vi "Write User Events.vi"(8 "error in (no error)":errorcluster, 10 "User Events to TCP Engine":T1, 11 "SLL Easy API via TCP in":refnum<class "SLL Easy API via TCP.lvclass">) -> (0 "error out":errorcluster, 3 "SLL Easy API via TCP out":refnum<class "SLL Easy API via TCP.lvclass">)   [LabVIEW 2016, in "SLL Easy API via TCP.lvclass"]
uses:
  SLL Easy API via TCP.lvclass
  _Typedefs/User Events to TCP Engine.ctl
  _Typedefs/TCP Event Data.ctl
  SLL Easy API via TCP.lvclass/SLL Easy API via TCP.ctl
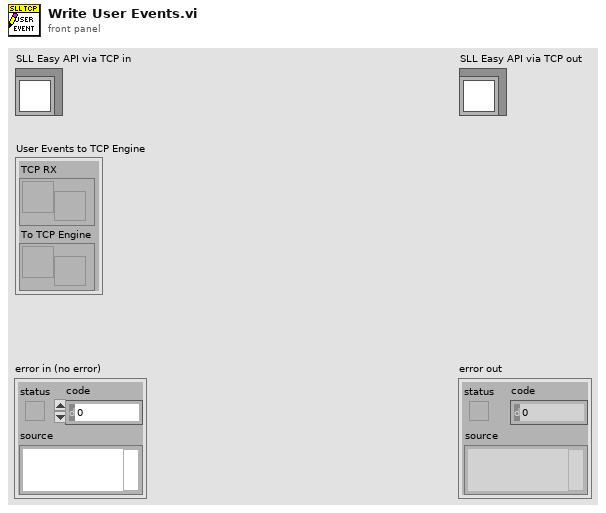
[diagram p1: front panel]
types:
  T1 = typedef "SLL Easy API via TCP.lvclass/User Events to TCP Engine.ctl" = cluster{"TCP RX":refnum<user-event>, "To TCP Engine":refnum<user-event>}
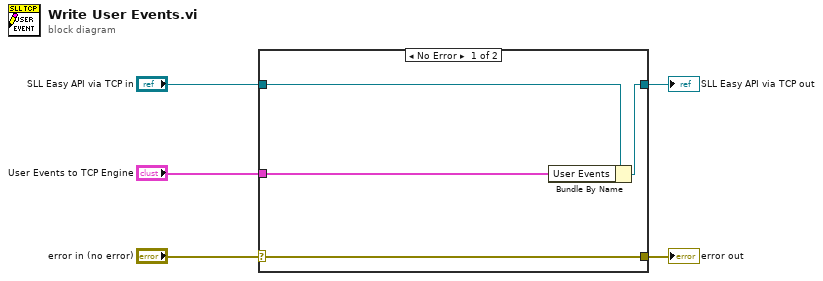
[diagram p0: block diagram]
diagram:
  n1 = case shown="No Error" "error in (no error)" {
    selector: "error in (no error)" -> [w9 w10]
    tunnel: [w9 w10] -> w4
    tunnel: [w7 w11] -> w2
    tunnel: "SLL Easy API via TCP in" -> [w8 w11]
    tunnel: "User Events to TCP Engine" -> [w6 _]
    frame No Error {
      n2 = Bundle By Name(cluster=w8, "User Events"=w6) -> (w7:refnum<class "SLL Easy API via TCP.lvclass">)
    }
    frame Error {
    }
  }
  "error out" <- w4
  "SLL Easy API via TCP out" <- w2
